vi "Solve Force.vi"(5 "I":dbl=1.0, 7 "E":dbl=1.0, 8 "y2":dbl, 9 "y1":dbl, 10 "x2":dbl, 11 "x1":dbl) -> (2 "D":dbl, 3 "P":dbl)   [LabVIEW 2015]
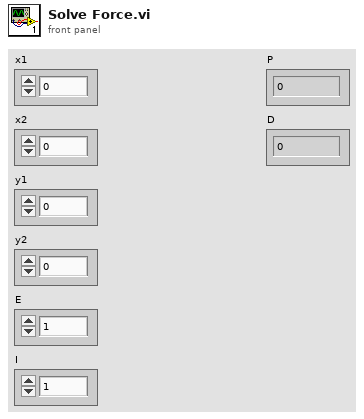
[diagram p1: front panel]
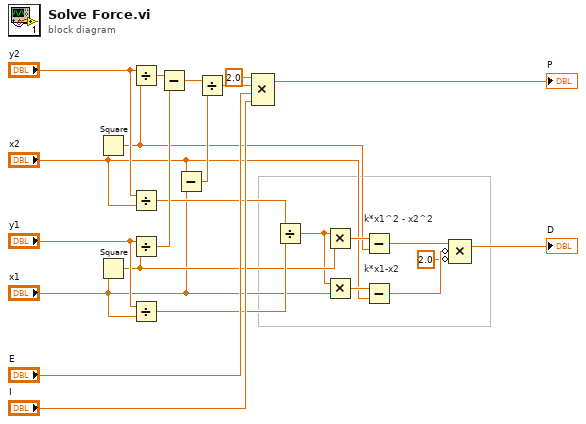
[diagram p0: block diagram]
diagram:
  n1 = Square(x="x2") -> (x^2=w9:dbl)
  n2 = Square(x="x1") -> (x^2=w11:dbl)
  n3 = Divide(x="y2", y=w9) -> (x/y=w24:dbl)
  n4 = Divide(x="y2", y="x2") -> (x/y=w13:dbl)
  n5 = Divide(x="y1", y=w11) -> (x/y=w23:dbl)
  n6 = Divide(x="y1", y="x1") -> (x/y=w12:dbl)
  n7 = Subtract(x=w24, y=w23) -> (x-y=w22:dbl)
  n8 = Subtract(x="x2", y="x1") -> (x-y=w21:dbl)
  n9 = Divide(x=w22, y=w21) -> (x/y=w20:dbl)
  n10 = Compound Arithmetic op=MULTIPLY(2.0 ("value"), w20, "E", "I") -> (→"P":dbl)
  n11 = Divide(x=w13, y=w12) -> (x/y=w8:dbl)
  n12 = Multiply(x=w8, y=w11) -> (x*y=w10:dbl)
  n13 = Multiply(x=w8, y="x1") -> (x*y=w6:dbl)
  n14 = Subtract "k*x1^2 - x2^2"(x=w10, y=w9) -> (x-y=w4:dbl)
  n15 = Subtract "k*x1-x2"(x=w6, y="x2") -> (x-y=w3:dbl)
  n16 = Compound Arithmetic op=MULTIPLY(w4, invert w3, invert 2.0 ("value")) -> (→"D":dbl)
